vi "New.vi"(0 "Invocation Request":refnum<class "Invocation Request ID.lvclass">, 5 "Arguments":string, 7 "ArgumentsKw":string="{}", 9 "Options":string="{}", 11 "error in (no error)":errorcluster) -> (4 "Yield JSON out":refnum<class "Yield JSON.lvclass">, 15 "error out":errorcluster)   [LabVIEW 2020, in "wamplv.lvlib" / "Yield JSON.lvclass"]
uses:
  Yield JSON.lvclass
  Yield JSON.lvclass/Yield JSON.ctl
  WAMP Client/Private/TypeDef/YIELD request data (JSON).ctl
  wamplv.lvlib
  Invocation Request ID/Invocation Request ID.lvclass
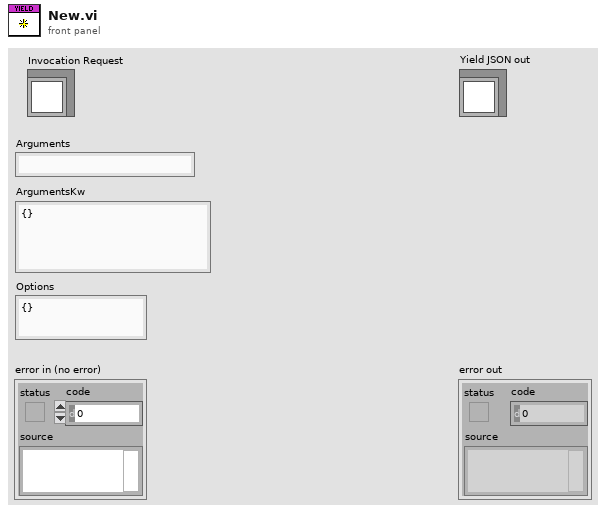
[diagram p1: front panel]
types:
  T1 = typedef "wamplv.lvlib/YIELD request data (JSON).ctl" = cluster{"Invocation Request ID":u64, "Arguments":string, "ArgumentsKw":string, "Options":string}
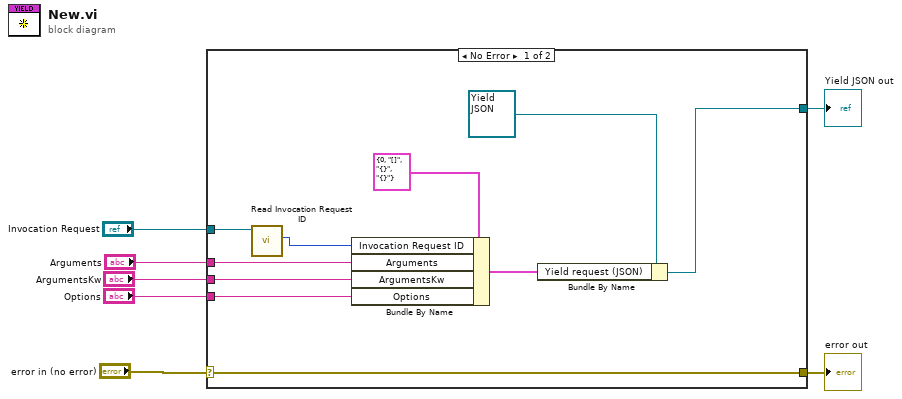
[diagram p0: block diagram]
diagram:
  n1 = case shown="No Error" "error in (no error)" {
    selector: "error in (no error)" -> [w17 w18]
    tunnel: [w17 w18] -> w6
    tunnel: [w8 _] -> w5
    tunnel: "Options" -> [w15 _]
    tunnel: "ArgumentsKw" -> [w14 _]
    tunnel: "Arguments" -> [w13 _]
    tunnel: "Invocation Request" -> [w12 _]
    frame No Error {
      n2 = call-dynamic "Read Invocation Request ID.vi"("Invocation Request in"=w12) -> ("Invocation Request ID"=w11:u64)  [unwired: 8 in, 2 out]
      n3 = Bundle By Name(cluster=T1 {"Invocation Request ID"=0, "Arguments"="[]", "ArgumentsKw"="{}", "Options"="{}"} ("Yield request"), "Invocation Request ID"=w11, "Arguments"=w13, "ArgumentsKw"=w14, "Options"=w15) -> (w9:T1)
      n4 = Bundle By Name(cluster=refnum<class "Yield JSON.lvclass"> refnum ("wamplv.lvlib:Yield JSON.lvclass"), "Yield request (JSON)"=w9) -> (w8:refnum<class "Yield JSON.lvclass">)
    }
    frame Error {
    }
  }
  "error out" <- w6
  "Yield JSON out" <- w5
